vi "params.To JSON Tree.vi"(8 "error in (no error)":errorcluster, 11 "params in":refnum<class "params.lvclass">) -> (0 "error out":errorcluster, 2 "JSON Value out":refnum<class "JSON Value.lvclass">, 3 "params out":refnum<class "params.lvclass">)   [LabVIEW 2016, in "params.lvclass"]
uses:
  params.lvclass
  <vilib>/NI/JSON Support for LabVIEW/JSON Value/JSON Value.lvclass
  params.lvclass/params.ctl
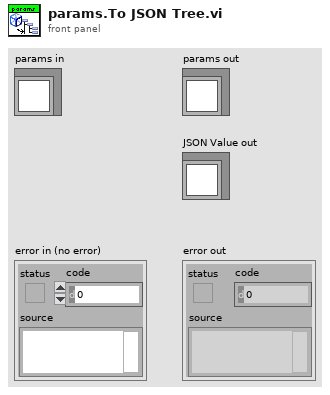
[diagram p1: front panel]
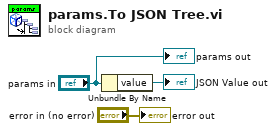
[diagram p0: block diagram]
diagram:
  n1 = Unbundle By Name("params in") -> ("value"=→"JSON Value out":refnum<class "JSON Value.lvclass">)
  "error out" <- "error in (no error)"
  "params out" <- "params in"
